vi "SVT Cross Spectrum (Mag-Phase).vi"(0 "scaled signal X [EUx]":waveform(dbl), 1 "scaled signal Y [EUy]":waveform(dbl), 2 "window":T10=1 items=["None"=0, "Hanning"=1, "Hamming"=2, "Blackman-Harris"=3, "Exact Blackman"=4, "Blackman"=5, "Flat Top"=6, "4 Term B-Harris "=7, "7 Term B-Harris"=8, "Low Sidelobe"=9, "Force - Exponential"=10, "Blackman Nuttall"=11, "Triangle"=30, "Bartlett-Hanning"=31, "Bohman"=32, "Parzen"=33, "Welch"=34, "Kaiser"=60, "Dolph-Chebyshev"=61, "Gaussian"=62], 4 "view":T8={"dB On (T)"=TRUE, "unwrap phase (F)"=FALSE, "convert to degree (T)"=TRUE}, 5 "error in (no error)":errorcluster, 7 "averaging parameters":T9={"averaging mode"=enum."No averaging", "weighting mode"=enum."Exponential", "number of averages"=10, "linear mode"=enum."One shot"}, 8 "force/exp settings":T7={"force window [%]"=50.0, "exp window [%]"=10.0} {"exp window [%]" min=0.0 max=100.0 format="%.2f"; "force window [%]" min=0.0 max=100.0 format="%.2f"}, 9 "restart averaging (F)":bool) -> (11 "averaging done":bool, 13 "averages completed":dbl, 14 "magnitude [dB EUx EUy]":cluster{"f0":dbl, "df":dbl, "magnitude":dbl[]} {"magnitude" format="%.2p"; "df" format="%.2p"; "f0" format="%.2p"}, 15 "magnitude unit label":string, 16 "phase [degrees]":cluster{"f0":dbl, "df":dbl, "phase":dbl[]} {"phase" format="%.2f"; "df" format="%.2f"; "f0" format="%.2f"}, 17 "phase unit label":string, 18 "spectrum info":T1={"channel name"="", "description"="", "x-axis units"=0, "spectral info"={"spectrum type"=enum."Power [Magnitude^2]", "linear/dB"=enum."linear", "window"=0, "window size"=0, "FFT size"=0}, "engineering units"=0, "custom label"="", "dB reference [EU]"=0.0, "peak units"=enum."rms", "weighting filter"=0, "spectral density?"=FALSE, "unit label"="", "spectrum skewed?"=FALSE, "complimentary spectrum units"=enum."none"} {"x-axis units" items=["Time (s)"=0, "Frequency-CB (Hz)"=1, "Frequency-CPB (Hz)"=1248, "Frequency-Arbitrary (Hz)"=2357, "Quefrency (s)"=2, "Revolutions (rev)"=3, "Order"=4, "Speed (RPM)"=11, "Speed (rad/s)"=21, "Index"=65535]; "weighting filter" items=["Linear", "A-weighting", "B-weighting", "C-weighting", "ITU-R 468-4", "Dolby", "CCITT", "C-message", "Wb", "Wc", "Wd", "We", "Wf", "Wh", "Wj", "Wk", "Wm", "AES17 20 kHz lowpass", "AES17 40 kHz lowpass", "AES17 20 kHz highpass", "AES17 40 kHz highpass"]; "dB reference [EU]" format="%.2f"; "engineering units" items=["custom..."=0, "V"=1, "A"=21, "C"=30, "pC"=31, "s"=32, "-"=29, "Pa"=2, "N"=20, "g"=3, "m/s^2"=4, "m/s"=5, "m"=6, "mm/s"=12, "mm"=13, "micron/s"=14, "micron"=15, "in/s^2"=7, "in/s"=8, "in"=9, "mil/s"=10, "mil"=11, "rad/s^2"=16, "rad/s"=17, "rad"=18, "deg/s^2"=26, "deg/s"=27, "deg"=28, "RPM"=22, "cycle/s^2"=23, "Hz"=24, "cycle"=25, "strain"=19]; "spectral info"."window" items=["None "=0, "Hanning"=1, "Hamming"=2, "Blackman-Harris"=3, "Exact Blackman"=4, "Blackman"=5, "Flat Top"=6, "4 Term B-Harris "=7, "7 Term B-Harris"=8, "Low Sidelobe"=9, "Force - Exponential"=10, "Gaussian"=62]}, 19 "error out":errorcluster)   [LabVIEW 2017]
doc: "Computes the cross power spectrum of <B>scaled signal X [EUx]</B> and <B>scaled signal Y [EUy]</B>. Results are returned in <B>magnitude [dB EUx EUy]</B> and <B>phase [degrees]</B>."
uses:
  <vilib>/addons/_NISVFA/_Shared subVIs/Controls/svc_Window [Dual FFT].ctl
  <vilib>/addons/_NISVFA/_Shared subVIs/Controls/svc_Spectrum Info.ctl
  <vilib>/addons/_NISVFA/_Shared subVIs/Controls/svc_X-Axis Units.ctl
  <vilib>/addons/_NISVFA/_Shared subVIs/Controls/svc_Spectrum Type.ctl
  <vilib>/addons/_NISVFA/_Shared subVIs/Controls/svc_Engineering Units Text Ring.ctl
  <vilib>/addons/_NISVFA/_Shared subVIs/Controls/svc_Weighting Filter Text Ring.ctl
  <vilib>/addons/_NISVFA/_Shared subVIs/Controls/svc_Complimentary Spectrum Units.ctl
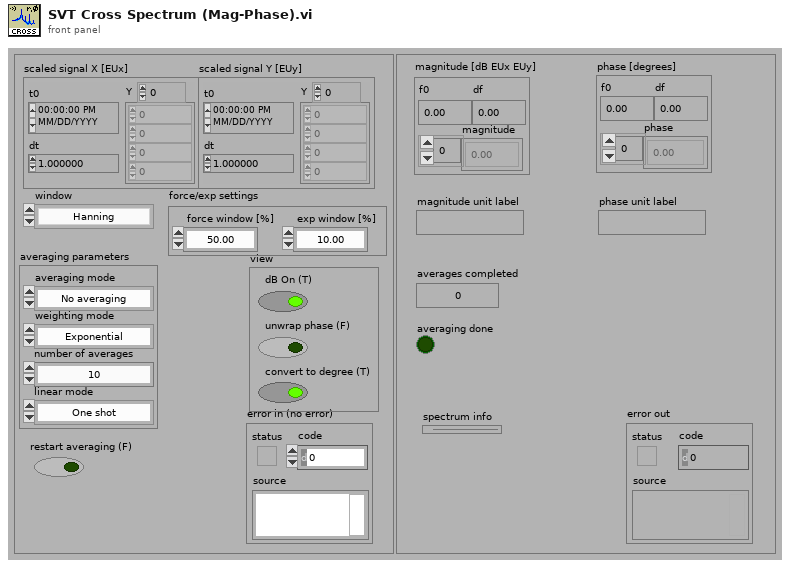
[diagram p1: front panel]
types:
  T1 = typedef "svc_Spectrum Info.ctl" = cluster{"channel name":string, "description":string, "x-axis units":T2, "spectral info":cluster{"spectrum type":T3, "linear/dB":enum16{"linear", "dB"}, "window":u16, "window size":i32, "FFT size":i32}, "engineering units":T4, "custom label":string, "dB reference [EU]":dbl, "peak units":enum16{"rms", "peak", "peak-peak"}, "weighting filter":T5, "spectral density?":bool, "unit label":string, "spectrum skewed?":bool, "complimentary spectrum units":T6}
  T2 = typedef "svc_X-Axis Units.ctl" = u16
  T3 = typedef "svc_Spectrum Type.ctl" = enum16{"FFT Spectrum [complex]", "Amplitude [Magnitude]", "Power [Magnitude^2]", "Cross Spectrum [complex]", "Frequency Response [Complex]"}
  T4 = typedef "svc_Engineering Units Text Ring.ctl" = u16
  T5 = typedef "svc_Weighting Filter Text Ring.ctl" = u16
  T6 = typedef "svc_Complimentary Spectrum Units.ctl" = enum16{"none", "radians", "degrees", "cycles", "imaginary"}
  T7 = cluster{"force window [%]":dbl, "exp window [%]":dbl}
  T8 = cluster{"dB On (T)":bool, "unwrap phase (F)":bool, "convert to degree (T)":bool}
  T9 = cluster{"averaging mode":enum16{"No averaging", "Vector averaging", "RMS averaging", "Peak hold"}, "weighting mode":enum16{"Linear", "Exponential"}, "number of averages":u32, "linear mode":enum16{"One shot", "Auto restart"}}
  T10 = typedef "svc_Window [Dual FFT].ctl" = u32
  T11 = enum16{"Cross spectrum", "Frequency response", "Coherent output power"}
  T12 = enum16{"Restart processing", "Continue processing", "Skip processing"}
  T13 = cluster{"f0":dbl, "df":dbl, "complex spectrum":cdb[]}
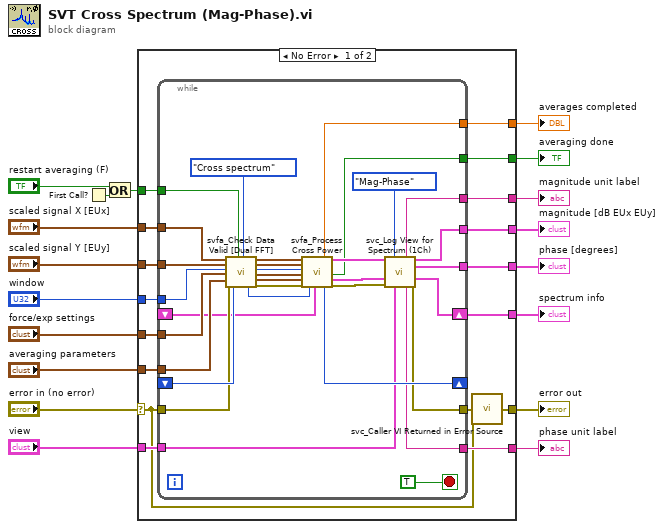
[diagram p0: block diagram]
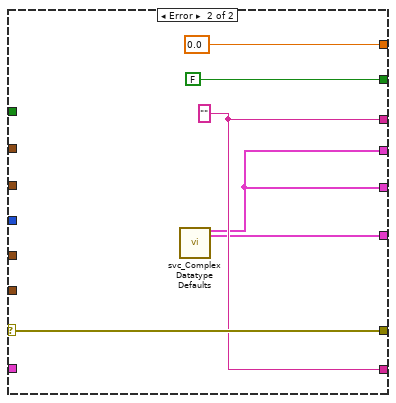
[diagram p2: hidden frame]
diagram:
  n1 = First Call?() -> (First Call?: T/F=w3:bool)
  n2 = Or(x="restart averaging (F)", y=w3) -> (x .or. y?=w1:bool)
  n3 = case shown="No Error" "error in (no error)" {
    selector: "error in (no error)" -> [w19 w73]
    tunnel: "window" -> [w30 _]
    tunnel: "averaging parameters" -> [w28 _]
    tunnel: "view" -> [w27 _]
    tunnel: [w20 w73] -> w15
    tunnel: [w23 w68] -> w14
    tunnel: [w24 w68] -> w13
    tunnel: "force/exp settings" -> [w29 _]
    tunnel: "scaled signal X [EUx]" -> [w32 _]
    tunnel: "scaled signal Y [EUy]" -> [w31 _]
    tunnel: w1 -> [w35 _]
    tunnel: [w26 w72] -> w8
    tunnel: [w25 w72] -> w7
    tunnel: [w33 0.0 ("averages completed")] -> w6
    tunnel: [w34 FALSE ("averaging done")] -> w5
    tunnel: [w22 w69] -> w4
    frame No Error {
      n4 = while {
        tunnel: [w39] -> w21
        tunnel: [w41] -> w23
        tunnel: [w42] -> w24
        tunnel: [w43] -> w25
        tunnel: [w44] -> w26
        tunnel: w27 -> [w46]
        tunnel: w19 -> [w47]
        tunnel: w28 -> [w48]
        tunnel: w29 -> [w49]
        tunnel: w30 -> [w50]
        tunnel: w31 -> [w51]
        tunnel: w32 -> [w52]
        tunnel: [w53] -> w33
        tunnel: [w54] -> w34
        shift-left: _ -> [w57]
        shift-right: [w55] -> _
        tunnel: w35 -> [w67]
        shift-right: [w40] -> w22
        shift-left: _ -> [w36]
        stop <- TRUE stop-if-true
        n5 = call <vilib>:"svfa_Check Data Valid [Dual FFT].vi"("stimulus [X]"=w52, "response [Y]"=w51, "window"=w50, "force/exp settings"=w49, "averaging parameters"=w48, "error in (no error)"=w47, "processing control in"=w57, "restart averaging (F)"=w67, "measurement"=T11."Cross spectrum") -> ("processing control out"=w56:T12, "dup stimulus [X]"=w65:waveform(dbl), "dup response [Y]"=w64:waveform(dbl), "window"=w63:T10, "dup force/exp settings"=w62:T7, "dup averaging parameters"=w61:T9, "error out"=w60:errorcluster)  [unwired: 3 in, 1 out]
        n6 = call <vilib>:"svfa_Process Cross Power.vi"("input signal X"=w65, "input signal Y"=w64, "window"=w63, "force/exp settings"=w62, "averaging parameters"=w61, "error in (no error)"=w60, "processing control in"=w56, "spectrum info in"=w36) -> ("averages completed"=w53:dbl, "processing control out"=w55:T12, "complex spectrum"=w59:T13, "averaging done"=w54:bool, "spectrum info out"=w37:T1, "error out"=w58:errorcluster)  [unwired: 6 in]
        n7 = call <vilib>:"svc_Log View for Spectrum (1Ch).vi"("complex spectrum"=w59, "View"=enum16{"Mag-Phase", "Real-Imaginary"}."Mag-Phase", "spectrum info in"=w37, "error in (no error)"=w58, "view"=w46) -> ("unit label [mag or real]"=w44:string, "magnitude or real"=w42:cluster{"f0":dbl, "df":dbl, dbl[]}, "phase or imag"=w41:cluster{"f0":dbl, "df":dbl, dbl[]}, "spectrum info out"=w40:T1, "unit label [phase or imag]"=w43:string, "error out"=w39:errorcluster)  [unwired: 5 in]
      }
      n8 = call <vilib>:"svc_Caller VI Returned in Error Source.vi"("warning input to caller"=w19, "error in (no error)"=w21) -> ("error out"=w20:errorcluster)  [unwired: 3 in]
    }
    frame Error {
      w72 = "" ("Unit label [Mag - Real]")
      n9 = call <vilib>:"svc_Complex Datatype Defaults.vi"() -> ("empty spectrum"=w68:cluster{"f0":dbl, "df":dbl, "magnitude":dbl[]}, "dead spectrum info"=w69:T1)  [unwired: 11 in, 7 out]
    }
  }
  "error out" <- w15
  "phase [degrees]" <- w14
  "magnitude [dB EUx EUy]" <- w13
  "magnitude unit label" <- w8
  "phase unit label" <- w7
  "averages completed" <- w6
  "averaging done" <- w5
  "spectrum info" <- w4
